vi "Cleanup Session.vi"(8 "error in (no error)":errorcluster, 11 "ADAS PE Template in":refnum<class "ADAS PE Template.lvclass">) -> (0 "error out":errorcluster, 3 "ADAS PE Template out":refnum<class "ADAS PE Template.lvclass">)   [LabVIEW 2020, in "ADAS PE Template.lvlib" / "ADAS PE Template.lvclass"]
doc: "<b>Cleanup Session</b>\nThis method is used to close any references opened in Configure Session and flush any buffers used.\n\nThis method is followed by either Configure Session (if the plugin is restarting) or Finalize (if the plugin is shutting down)."
uses:
  ADAS PE Template.lvclass
  C:/Program Files/National Instruments/LabVIEW 2020/vi.lib/FlexLogger/SDK/PluginSDK.lvlibp/PEFClasses/SDK/Processing Element/Processing Element.lvclass
  <vilib>/FlexLogger/SDK/PluginSDK.lvlibp/PEFClasses/SDK/Processing Element/Read Alias.vi
  <vilib>/ADAS Record/pefCommon/Tracing/SendGenericEvent.vi
  ADAS PE Template.lvclass/ADAS PE Template.ctl
  <vilib>/ADAS Record/Utilities/ADAS Utilities.lvlib
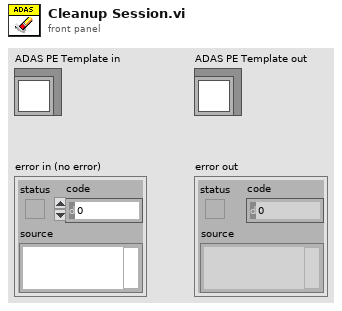
[diagram p1: front panel]
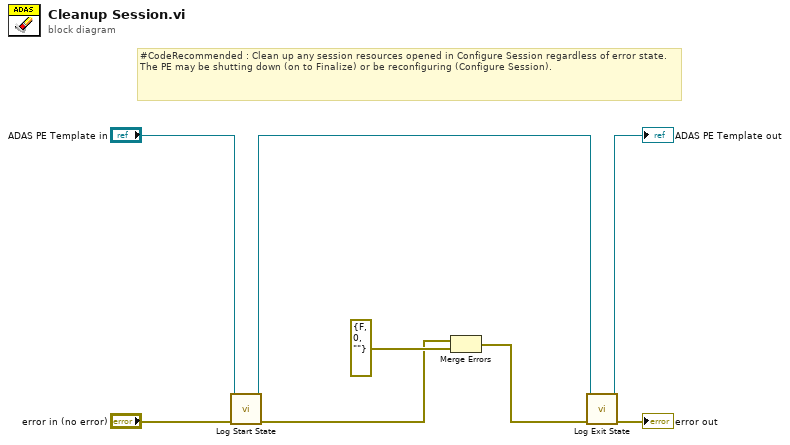
[diagram p0: block diagram]
diagram:
  # "#CodeRecommended : Clean up any session resources opened in Configure Session regardless of error state. The PE may be shutting down (on to Finalize) or be reconfiguring (Configure Session)."
  n1 = call <vilib>:"Log Start State.vi"("error in (no error)"="error in (no error)", "PluginSDK.lvlibp:Processing Element.lvclass"="ADAS PE Template in") -> ("error out"=w6:errorcluster, "PluginSDK.lvlibp:Processing Element.lvclass"=w2:refnum<class "ADAS PE Template.lvclass">)  [unwired: 8 in]
  n2 = Merge Errors(w6, errorcluster {"status"=FALSE, "code"=0, "source"=""} ("error in")) -> (w4:errorcluster)
  n3 = call <vilib>:"Log Exit State.vi"("error in (no error)"=w4, "PluginSDK.lvlibp:Processing Element.lvclass"=w2) -> ("error out"=→"error out":errorcluster, "PluginSDK.lvlibp:Processing Element.lvclass"=→"ADAS PE Template out":refnum<class "ADAS PE Template.lvclass">)  [unwired: 8 in]
